vi "Static.Generate.Digital.vi"(11 "Settings":T1={"ACTIVE EDGE"=TRUE, "OUTPUT"=FALSE}) -> (3 "Output":bool)   [LabVIEW 2015, in "Speciality FPGA IO.lvlib"]
uses:
  Speciality FPGA IO.lvlib
  Types/Static.Generate.Digital.Settings.ctl
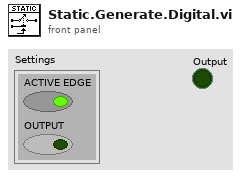
[diagram p1: front panel]
types:
  T1 = typedef "Speciality FPGA IO.lvlib/Static.Generate.Digital.Settings.ctl" = cluster{"ACTIVE EDGE":bool, "OUTPUT":bool}
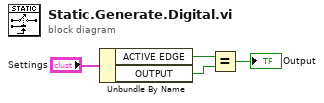
[diagram p0: block diagram]
diagram:
  n1 = Unbundle By Name("Settings") -> ("ACTIVE EDGE"=w3:bool, "OUTPUT"=w2:bool)
  n2 = Equal?(x=w3, y=w2) -> (x = y?=→"Output":bool)
